vi "Query Steps.vi"() -> ()   [LabVIEW 2024]
uses:
  <vilib>/Plug-In SDKs/Clients/Data Store V1/Data Store Client.lvlibp
panel:
  out "queried steps":string[](array[string])
  in  "odata query":string="$filter=contains(Name,'Voltage')"
  out "error out":errorcluster
  # "Query Steps\n\nThis VI provides examples of querying Step items.\nRun Publish Data.vi to create data to query with this VI."
  # "To query all steps, specify a blank string for 'odata query'."
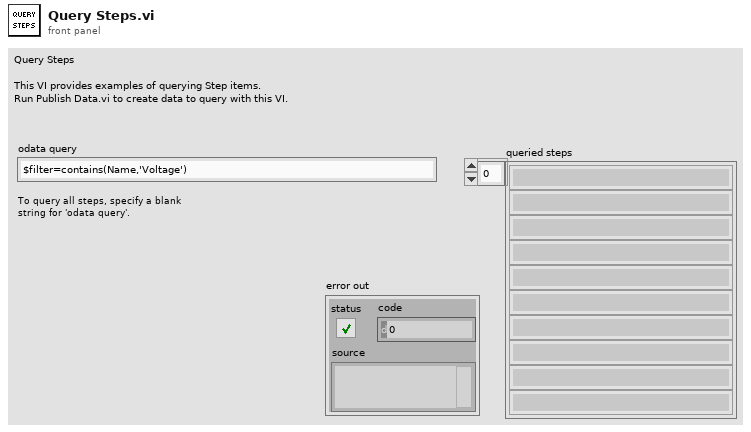
[diagram p1: front panel]
types:
  T1 = typedef "NI Metadata Types.lvlib/Step.ctl" = cluster{"step name":string, "step type":string, "start date time":timestamp, "end date time":timestamp, "notes":string, "step id":string, "parent step id":string, "test result id":string, "test id":string, "link":string, "extensions":T2[], "schema id":string}
  T2 = typedef "NI Metadata Types.lvlib/Extension.ctl" = cluster{"name":string, "value":string}
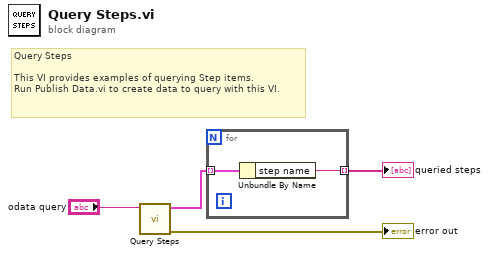
[diagram p0: block diagram]
diagram:
  # "Query Steps\n\nThis VI provides examples of querying Step items.\nRun Publish Data.vi to create data to query with this VI."
  n1 = call <vilib>:"Query Steps.vi"("odata query"="odata query") -> ("error out"=→"error out":errorcluster, "steps"=w3:T1[])  [unwired: 9 in]
  n2 = for {
    tunnel: w3 -> [w6] mode=indexing
    tunnel: [w5] -> w1 mode=indexing
    n3 = Unbundle By Name(w6) -> ("step name"=w5:string)
  }
  "queried steps" <- w1
